vi "RecordAV_CB.vi"(4 "ErrorIn":errorcluster, 5 "DataFolder":string="00000000-000000", 6 "Source":enum16{"AI0", "SoundCard"}(ring), 7 "Mode":T2(ring)=enum."Close") -> (0 "ErrorOut":errorcluster={"status"=FALSE, "code"=209801, "source"="Send2Grapevine32.vi"})   [LabVIEW 2013]
doc: "The Low-Level Grab VI configures the number of buffers to use for the acquisition and configures an event callback to handle every other acquired image. A grab is appropriate for high-speed applications in which you need to process only one image at a time."
uses:
  <vilib>/vision/Image Controls.llb/IMAQ Image.ctl
  <vilib>/userdefined/High Color/IMAQdx.ctl
  <vilib>/vision/Avi.llb/IMAQ AVI2 Refnum.ctl
  <vilib>/sound2/lvsound2.llb/Sound File Refnum.ctl
  <vilib>/sound2/lvsound2.llb/Sound Input Task ID.ctl
  <vilib>/vision/driver/IMAQdx.llb/IMAQdx Acquisition Mode.ctl
  <vilib>/sound2/lvsound2.llb/Sound Data Format.ctl
  <vilib>/sound2/lvsound2.llb/Sampling Mode.ctl
  <vilib>/vision/driver/IMAQdx.llb/IMAQdx Buffer Number Mode.ctl
  <vilib>/DAQmx/read.llb/DAQmx Read (Analog 2D DBL NChan NSamp).vi
  <vilib>/sound2/lvsound2.llb/Sound File Write Open.vi
  <vilib>/sound2/lvsound2.llb/Sound File Write (DBL Single).vi
  Globals.vi
  <vilib>/DAQmx/miscellaneous.llb/DAQmx Fill In Error Info.vi
  <vilib>/sound2/lvsound2.llb/Sound Input Read (SGL).vi
  <vilib>/vision/driver/NI_Vision_Acquisition_Software.lvlib
  <resource>/objmgr/imaqdx.rc
panel:
  out "iSource":enum16{"AI0", "SoundCard"}(ring)=enum."SoundCard"
  out "AudID":T1=1 format="%.0x"
  out "VidTask":T3="cam1"
  out "AudTask":refnum<k21>
  out "WAVRef":T4
  out "AVIRef":T5
  out "FrmEvnt":refnum<event-registration>
  out "BufferImg":T6
  out "StopAud":bool
  out "StopVid":bool
  out "StitchResult":string="ffmpeg version N-51683-g9dc88ac Copyright (c) 2000-2013 the FFmpeg developers\r\n  built on Apr  8 2013 21:24:37 with gcc 4.8.0 (GCC)\r\n  configuration: --enable-gpl --enable-version3 --disable-w32threads --enable-avisynth --enable-bzlib --enable-fontconfig --enable-frei0r --enable-gnutls --enable-iconv --enable-libass --enable-libbluray --enable-libcaca --enable-libfreetype --enable-libgsm --enable-libilbc --enable-libmp3lame --enable-libopencore-amrnb --enable-libopencore-amrwb --enable-libopenjpeg --enable-libopus --enable-librtmp --enable-libschroedinger --enable-libsoxr --enable-libspeex --enable-libtheora --enable-libtwolame --enable-libvo-aacenc --enable-libvo-amrwbenc --enable-libvorbis --enable-libvpx --enable-libx264 --enable-libxavs --enable-libxvid --enable-zlib\r\n  libavutil      52. 25.100 / 52. 25.100\r\n  libavcodec     55.  2.100 / 55.  2.100\r\n  libavformat    55.  1.100 / 55.  1.100\r\n  libavdevice    55.  0.100 / 55.  0.100\r\n  libavfilter     3. 49.101 /  3. 49.101\r\n  libswscale      2.  2.100 /  2.  2.100\r\n  libswresample   0. 17.102 /  0. 17.102\r\n  libpostproc    52.  2.100 / 52.  2.100\r\nInput #0, avi, from 'D:\\20140505-075330\\20140505-075330.avi':\r\n  Duration: 00:00:50.56, start: 0.000000, bitrate: 1016 kb/s\r\n    Stream #0:0: Video: mpeg4 (Simple Profile) (XVID / 0x44495658), yuv420p, 1280x720 [SAR 1:1 DAR 16:9], 25 tbr, 25 tbn, 25 tbc\r\n[wav @ 0000000003b3a5a0] max_analyze_duration 5000000 reached at 5015510 microseconds\r\nGuessed Channel Layout for  Input Stream #1.0 : mono\r\nInput #1, wav, from 'D:\\20140505-075330\\20140505-075330.wav':\r\n  Duration: 00:00:50.00, bitrate: 705 kb/s\r\n    Stream #1:0: Audio: pcm_s16le ([1][0][0][0] / 0x0001), 44100 Hz, mono, s16, 705 kb/s\r\nOutput #0, avi, to 'D:\\20140505-075330\\20140505-075330_Mixed.avi':\r\n  Metadata:\r\n    ISFT            : Lavf55.1.100\r\n    Stream #0:0: Video: mpeg4 (XVID / 0x44495658), yuv420p, 1280x720 [SAR 1:1 DAR 16:9], q=2-31, 25 tbn, 25 tbc\r\n    Stream #0:1: Audio: mp3 (U[0][0][0] / 0x0055), 44100 Hz, mono, s16p\r\nStream mapping:\r\n  Stream #0:0 -> #0:0 (copy)\r\n  Stream #1:0 -> #0:1 (pcm_s16le -> libmp3lame)\r\nPress [q] to stop, [?] for help\r\nframe=  184 fps=0.0 q=-1.0 size=     434kB time=00:00:07.36 bitrate= 482.9kbits/s    \rframe=  738 fps=726 q=-1.0 size=    4068kB time=00:00:29.52 bitrate=1129.0kbits/s    \rframe= 1264 fps=1015 q=-1.0 Lsize=    6718kB time=00:00:50.56 bitrate=1088.5kbits/s    \r\r\nvideo:6241kB audio:391kB subtitle:0 global headers:0kB muxing overhead 1.308708%\r\n"
  out "WAVName":path=path "D:/20140505-075330/20140505-075330.wav"
  out "AVIName":path=path "D:/20140505-075330/20140505-075330.avi"
  out "FrameRate":dbl=25.0
  out "WAVChart":dbl[](graph)=[0.01885986328125, 0.02471923828125, 0.026458740234375, 0.019622802734375, 0.015625, 0.016571044921875, 0.017852783203125, 0.016937255859375, 0.02349853515625, 0.0262451171875, 0.021697998046875, 0.01995849609375, 0.013427734375, 0.008819580078125, 0.013916015625, 0.016693115234375, 0.0172119140625, 0.023468017578125, 0.0235595703125, 0.018890380859375, 0.022369384765625, 0.022003173828125, 0.019378662109375, 0.017578125, 0.0115966796875, 0.011688232421875, 0.011016845703125, 0.007659912109375, 0.012359619140625, 0.015167236328125, 0.010162353515625, 0.00787353515625, 0.010009765625, 0.01434326171875, 0.018524169921875, 0.019012451171875, 0.019317626953125, 0.019500732421875, 0.021514892578125, 0.021514892578125, 0.0233154296875, 0.02276611328125, 0.0174560546875, 0.018585205078125, 0.019439697265625, 0.01959228515625, 0.0185546875, 0.015594482421875, 0.01593017578125, 0.0162353515625, 0.013427734375, 0.01519775390625, 0.005340576171875, 0.008026123046875, 0.00811767578125, 0.004669189453125, 0.008148193359375, 0.00384521484375, 0.007598876953125, 0.007354736328125, 0.009735107421875, 0.01580810546875, 0.01385498046875, 0.014923095703125, 0.00830078125, 0.005096435546875, 0.008941650390625, 0.01416015625, 0.01220703125, 0.0140380859375, 0.01275634765625, 0.006439208984375, 0.007049560546875, 0.006134033203125, -0.000457763671875, 0.003326416015625, 0.0081787109375, 0.009124755859375, 0.013458251953125, 0.014007568359375, 0.014312744140625, 0.006011962890625, 0.00238037109375, 0.010284423828125, 0.011962890625, 0.009857177734375, 0.00909423828125, 0.016448974609375, 0.01885986328125, 0.01190185546875, 0.010955810546875, 0.01019287109375, 0.00152587890625, 0.00762939453125, 0.008270263671875, 0.00604248046875, 0.010589599609375, 0.0037841796875, 0.0050048828125, 0.007080078125, 0.004669189453125, 0.0064697265625, 0.01068115234375, 0.009521484375, 0.002532958984375, -0.000518798828125, 0.005035400390625, 0.0042724609375, 0.00164794921875, 0.0001220703125, -0.002716064453125, -0.00164794921875, -0.007232666015625, -0.01153564453125, -0.005889892578125, -0.00341796875, -0.008514404296875, -0.007415771484375, -0.00726318359375, -0.007781982421875, -0.009918212890625, -0.010772705078125, -0.00628662109375, -0.001373291015625, -0.0008544921875, -0.003997802734375, 0.003021240234375, 0.003082275390625, 0.000640869140625, 0.00250244140625, 0.002960205078125, 0.00115966796875, 0.000579833984375, -0.002166748046875, -0.00115966796875, -0.006591796875, -0.0128173828125, -0.013275146484375, -0.0157470703125, -0.016204833984375, -0.013885498046875, -0.01531982421875, -0.00897216796875, -0.00762939453125, -0.00738525390625, -0.00311279296875, -0.002166748046875, 0.000244140625, -0.003509521484375, -0.003662109375, 0.001220703125, 0.001251220703125, 0.0001220703125, -0.003692626953125, -0.003997802734375, -0.004364013671875, -9.1552734375e-05, 0.00341796875, 0.000457763671875, -0.000274658203125, -0.0006103515625, 0.00543212890625, 0.001312255859375, 0.003662109375, 0.009765625, 0.004852294921875, 0.003997802734375, 0.00189208984375, -0.000213623046875, -0.006500244140625, -0.006744384765625, -0.0120849609375, -0.012359619140625, -0.003631591796875, -0.005645751953125, -0.0028076171875, 0.00286865234375, -0.00311279296875, -0.005279541015625, 0.001922607421875, -0.003753662109375, -0.000335693359375, -0.00299072265625, 0.001556396484375, 0.00299072265625, 0.006317138671875, 0.006622314453125, -0.003692626953125, -0.007110595703125, 0.001190185546875, -0.002288818359375, 0.00030517578125, 0.007720947265625, 0.003692626953125, 0.006011962890625, 0.007904052734375, 0.0115966796875, 0.01513671875, 0.00421142578125, 0.00299072265625, 0.002532958984375, 0.0009765625, 0.0018310546875, 0.001556396484375, 0.00640869140625, 0.008148193359375, 0.011962890625, 0.01416015625, 0.01055908203125, 0.0126953125, 0.006500244140625, 0.00958251953125, 0.009613037109375, 0.00921630859375, 0.007049560546875, 0.00927734375, 0.011871337890625, 0.015655517578125, 0.0146484375, 0.011627197265625, 0.0162353515625, 0.007965087890625, 0.00146484375, 0.004425048828125, 0.007415771484375, 0.007598876953125, 0.011810302734375, 0.01324462890625, 0.016357421875, 0.0126953125, 0.012451171875, 0.01763916015625, 0.0196533203125, 0.019775390625, 0.021453857421875, 0.025848388671875, 0.023468017578125, 0.01934814453125, 0.019073486328125, 0.020355224609375, 0.021270751953125, 0.024139404296875, 0.02545166015625, 0.0255126953125, 0.027862548828125, 0.027435302734375, 0.030487060546875, 0.029052734375, 0.032196044921875, 0.030120849609375, 0.035552978515625, 0.026611328125, 0.025787353515625, 0.030303955078125, 0.021270751953125, 0.027099609375, 0.032379150390625, 0.03143310546875, 0.02508544921875, 0.03118896484375, 0.029510498046875, 0.0311279296875, 0.03460693359375, 0.0340576171875, 0.027435302734375, 0.03076171875, 0.031707763671875, 0.029815673828125, 0.0341796875, 0.039337158203125, 0.0396728515625, 0.039459228515625, 0.031463623046875, 0.025482177734375, 0.03057861328125, 0.031707763671875, 0.03253173828125, 0.035308837890625, 0.0355224609375, 0.035369873046875, 0.02996826171875, 0.0267333984375, 0.025665283203125, 0.024688720703125, 0.029754638671875, 0.023681640625, 0.02490234375, 0.026458740234375, 0.025726318359375, 0.03436279296875, 0.028411865234375, 0.0225830078125, 0.02349853515625, 0.021270751953125, 0.02691650390625, 0.02520751953125, 0.023101806640625, 0.020782470703125, 0.0198974609375, 0.024200439453125, 0.021148681640625, 0.023406982421875, 0.028289794921875, 0.02862548828125, 0.03240966796875, 0.025634765625, 0.030120849609375, 0.029998779296875, 0.02752685546875, 0.033660888671875, 0.028167724609375, 0.032073974609375, 0.033233642578125, 0.02862548828125, 0.029876708984375, 0.02667236328125, 0.02392578125, 0.02764892578125, 0.026275634765625, 0.023468017578125, 0.031158447265625, 0.0306396484375, 0.022125244140625, 0.022430419921875, 0.025054931640625, 0.02337646484375, 0.025299072265625, 0.02777099609375, 0.03326416015625, 0.02777099609375, 0.025390625, 0.028778076171875, 0.02239990234375, 0.01837158203125, 0.021148681640625, 0.021514892578125, 0.018218994140625, 0.01593017578125, 0.017547607421875, 0.018524169921875, 0.01739501953125, 0.01922607421875, 0.016632080078125, 0.010772705078125, 0.013519287109375, 0.011383056640625, 0.013671875, 0.017242431640625, 0.021636962890625, 0.01922607421875, 0.01593017578125, 0.016571044921875, 0.015777587890625, 0.016693115234375, 0.011260986328125, 0.005828857421875, 0.0068359375, 0.001739501953125, 0.00518798828125, 0.006591796875, 0.00286865234375, 0.015289306640625, 0.011383056640625, 0.01031494140625, 0.00927734375, 0.009307861328125, 0.011199951171875, 0.010894775390625, 0.006927490234375, 0.0115966796875, 0.004638671875, 0.004425048828125, 0.003631591796875, 0.007659912109375, 0.0086669921875, 0.00616455078125, 0.003509521484375, -0.000518798828125, 0.0001220703125, -0.001708984375, -0.0015869140625, 0.002349853515625, 0.0089111328125, 0.007171630859375, 0.0072021484375, 0.004791259765625, 0.00341796875, 0.001068115234375, 0.00341796875, 0.00445556640625, 0.008056640625, 0.009246826171875, 0.011077880859375, 0.006195068359375, 0.005340576171875, 0.00244140625, 0.006561279296875, 0.016021728515625, 0.011322021484375, 0.0079345703125, 0.006622314453125, 0.01080322265625, 0.009796142578125, 0.0028076171875, 0.00439453125, 0.00048828125, 0.0052490234375, 0.0025634765625, 0.00396728515625, 0.0057373046875, 0.00860595703125, 0.00701904296875, 0.0020751953125, -0.00189208984375, -0.001861572265625, 0.00091552734375, -0.00762939453125, -0.0074462890625, -0.0054931640625, 0.0010986328125, 0.00421142578125, 0.001800537109375, 0.007232666015625, -0.001190185546875, 9.1552734375e-05, -0.0078125, -0.010833740234375, -0.0068359375, -0.0054931640625, -0.004791259765625, -0.011016845703125, -0.009765625, -0.007720947265625, -0.00384521484375, -0.011260986328125, -0.00848388671875, -0.000152587890625, -0.00030517578125, -0.00177001953125, -0.0052490234375, -0.00994873046875, -0.001617431640625, -0.00567626953125, -0.008209228515625, -0.004638671875, -0.0057373046875, -0.0067138671875, -0.01080322265625, -0.008544921875, -0.0120849609375, -0.009857177734375, -0.01409912109375, -0.0184326171875, -0.022003173828125, -0.023101806640625, -0.02197265625, -0.021942138671875, -0.018035888671875, -0.016632080078125, -0.025726318359375, -0.032623291015625, -0.02557373046875, -0.03179931640625, -0.020660400390625, -0.017578125, -0.01641845703125, -0.017852783203125, -0.02423095703125, -0.030609130859375, -0.03009033203125, -0.027862548828125, -0.031646728515625, -0.03076171875, -0.0225830078125, -0.015472412109375, -0.018341064453125, -0.02520751953125, -0.032958984375, -0.034759521484375, -0.034637451171875, -0.033233642578125, -0.031768798828125, -0.025238037109375, -0.02752685546875, -0.03057861328125, -0.0286865234375, -0.03204345703125, -0.02850341796875, -0.020965576171875, -0.022735595703125, -0.02435302734375, -0.024383544921875, -0.02496337890625, -0.01910400390625, -0.0230712890625, -0.0225830078125, -0.02435302734375, -0.027984619140625, -0.027740478515625, -0.026153564453125, -0.03021240234375, -0.030792236328125, -0.0277099609375, -0.0250244140625, -0.02239990234375, -0.025146484375, -0.029571533203125, -0.022491455078125, -0.02587890625, -0.02081298828125, -0.024688720703125, -0.026885986328125, -0.026214599609375, -0.025482177734375, -0.027374267578125, -0.03387451171875, -0.03570556640625, -0.0379638671875, -0.03662109375, -0.034637451171875, -0.03826904296875, -0.0408935546875, -0.037384033203125, -0.038177490234375, -0.039337158203125, -0.03564453125, -0.02972412109375, -0.02410888671875, -0.01873779296875, -0.02288818359375, -0.02679443359375, -0.03839111328125, -0.0316162109375, -0.029449462890625, -0.02972412109375, -0.03564453125, -0.034332275390625, -0.038665771484375, -0.044525146484375, -0.040374755859375, -0.039031982421875, -0.03741455078125, -0.039703369140625, -0.0386962890625, -0.036834716796875, -0.03521728515625, -0.033905029296875, -0.02984619140625, -0.035430908203125, -0.032440185546875, -0.029022216796875, -0.024688720703125, -0.024139404296875, -0.027099609375, -0.027313232421875, -0.02496337890625, -0.02203369140625, -0.0244140625, -0.021240234375, -0.02392578125, -0.020782470703125, -0.01873779296875, -0.0208740234375, -0.0208740234375, -0.022491455078125, -0.01806640625, -0.0216064453125, -0.017181396484375, -0.01397705078125, -0.01556396484375, -0.009979248046875, -0.016693115234375, -0.01068115234375, -0.016754150390625, -0.01959228515625, -0.016143798828125, -0.02447509765625, -0.029266357421875, -0.026947021484375, -0.02496337890625, -0.0345458984375, -0.027618408203125, -0.0318603515625, -0.028656005859375, -0.02685546875, -0.025634765625, -0.02392578125, -0.026031494140625, -0.014617919921875, -0.018585205078125, -0.021697998046875, -0.019317626953125, -0.02044677734375, -0.0184326171875, -0.018951416015625, -0.022125244140625, -0.019073486328125, -0.02203369140625, -0.0224609375, -0.02166748046875, -0.019073486328125, -0.015411376953125, -0.016448974609375, -0.023834228515625, -0.021728515625, -0.016387939453125, -0.009490966796875, -0.012542724609375, -0.0169677734375, -0.017822265625, -0.02105712890625, -0.017913818359375, -0.016815185546875, -0.01983642578125, -0.0179443359375, -0.0123291015625, -0.01129150390625, -0.01324462890625, -0.015869140625, -0.01385498046875, -0.016387939453125, -0.015655517578125, -0.0181884765625, -0.017578125, -0.013092041015625, -0.008331298828125, -0.007781982421875, -0.00439453125, -0.007080078125, -0.010223388671875, -0.01239013671875, -0.014923095703125, -0.01080322265625, -0.001983642578125, -0.0074462890625, -0.017791748046875, -0.023040771484375, -0.02978515625, -0.0267333984375, -0.0224609375, -0.017120361328125, -0.024871826171875, -0.01788330078125, -0.012298583984375, -0.011566162109375, -0.00726318359375, -0.00457763671875, -0.00299072265625, 0.00146484375, -0.0037841796875, -0.008819580078125, -0.0076904296875, -0.006256103515625, 0.001373291015625, -0.001708984375, -0.00335693359375, 0.001953125, 0.005859375, 0.00396728515625, 0.007110595703125, 0.011993408203125, 0.005828857421875, 0.00677490234375, 0.000244140625, 0.008575439453125, 0.0098876953125, 0.003875732421875, 0.0067138671875, 0.000946044921875, 0.00274658203125, 0.001800537109375, 0.00506591796875, 0.006072998046875, -0.006103515625, -0.00909423828125, -0.003936767578125, -0.001861572265625, -0.002777099609375, 0.001495361328125, 0.0006103515625, -0.003265380859375, -0.0003662109375, 0.00128173828125, 0.0010986328125, 0.002655029296875, -0.005615234375, -0.01275634765625, -0.00775146484375, -0.004913330078125, -0.004119873046875, -0.00506591796875, -9.1552734375e-05, 0.003204345703125, -0.002410888671875, -0.001800537109375, 0.001312255859375, 0.003173828125, -0.002899169921875, -0.004608154296875, 0.002593994140625, -0.002685546875, -0.00762939453125, -0.0028076171875, -0.006805419921875, -0.0146484375, -0.009979248046875, -0.00177001953125, 0.00286865234375, -0.0091552734375, -0.01495361328125, -0.01080322265625, -0.009368896484375, 0.0023193359375, -0.0010986328125, -0.001678466796875, -0.00177001953125, -0.006134033203125, -0.004730224609375, -0.00921630859375, -0.00909423828125, -0.0108642578125, -0.017181396484375, -0.015289306640625, -0.01458740234375, -0.013336181640625, -0.0057373046875, -0.004852294921875, -0.005645751953125, -0.0050048828125, -0.006500244140625, -0.00927734375, -0.012908935546875, -0.014404296875, -0.0155029296875, -0.0115966796875, -0.009796142578125, -0.01202392578125, -0.018157958984375, -0.021240234375, -0.015533447265625, -0.01629638671875, -0.01318359375, -0.015594482421875, -0.020721435546875, -0.017974853515625, -0.02056884765625, -0.02264404296875, -0.01654052734375, -0.01702880859375, -0.0146484375, -0.013275146484375, -0.023040771484375, -0.015960693359375, -0.013092041015625, -0.011077880859375, -0.009063720703125, -0.01727294921875, -0.018035888671875, -0.01580810546875, -0.011932373046875, -0.01287841796875, -0.003692626953125, -0.015167236328125, -0.014068603515625, -0.01666259765625, -0.0211181640625, -0.01812744140625, -0.013336181640625, -0.01519775390625, -0.0093994140625, -0.012847900390625, -0.0208740234375, -0.01300048828125, -0.006988525390625, -0.006072998046875, -0.011199951171875, -0.01263427734375, -0.01263427734375, -0.015625, -0.01055908203125, -0.00372314453125, -0.001312255859375, 0.001861572265625, -6.103515625e-05, -0.00311279296875, -0.001251220703125, -0.006500244140625, -0.00665283203125, 0.000823974609375, 0.001190185546875, 0.004486083984375, -0.004638671875, -0.00250244140625, -0.000518798828125, 0.001739501953125, 0.010955810546875, 0.00384521484375, -0.002349853515625, -0.00128173828125, -0.002227783203125, -0.005157470703125, -0.003204345703125, -0.00482177734375, -0.006072998046875, -0.001312255859375, -0.00018310546875, 0.0001220703125, -0.000274658203125, 0.003753662109375, 0.0103759765625, 0.009063720703125, 0.01324462890625, 0.019989013671875, 0.01324462890625, 0.015350341796875, 0.017791748046875, 0.019744873046875, 0.0157470703125, 0.007049560546875, 0.01263427734375, 0.0111083984375, 0.009002685546875, 0.01141357421875, 0.016632080078125, 0.012847900390625, 0.007568359375, 0.0042724609375, -0.00372314453125, -0.011383056640625, 0.00128173828125, 0.014312744140625, 0.016082763671875, 0.021697998046875, 0.020172119140625, 0.021575927734375, 0.02032470703125, 0.02215576171875, 0.02471923828125, 0.0302734375, 0.02752685546875, 0.02667236328125, 0.026580810546875, 0.0250244140625, 0.027557373046875, 0.020172119140625, 0.0247802734375, 0.02978515625, 0.030120849609375, 0.03131103515625, 0.031524658203125, 0.032257080078125, 0.0286865234375, 0.03033447265625, 0.0279541015625, 0.03582763671875, 0.036285400390625, 0.03515625, 0.028656005859375, 0.0311279296875, 0.033599853515625, 0.03582763671875, 0.028839111328125, 0.02947998046875, 0.0306396484375, 0.025146484375, 0.020843505859375, 0.027679443359375, 0.028045654296875, 0.02532958984375, 0.024017333984375, 0.02410888671875, 0.032073974609375, 0.018951416015625, 0.02801513671875, 0.0318603515625, 0.02587890625, 0.02825927734375, 0.025421142578125, 0.033203125, 0.03515625, 0.0362548828125, 0.030975341796875, 0.034332275390625, 0.02392578125, 0.027191162109375, 0.03472900390625, 0.03515625, 0.02813720703125, 0.0291748046875, 0.028717041015625, 0.027099609375, 0.02874755859375, 0.02203369140625, 0.019805908203125, 0.0179443359375, 0.0289306640625, 0.023773193359375, 0.017059326171875, 0.020904541015625, 0.0262451171875, 0.022979736328125, 0.021453857421875, 0.024017333984375, 0.02056884765625, 0.022430419921875, 0.02081298828125, 0.021759033203125, 0.026611328125, 0.033660888671875, 0.027374267578125, 0.02435302734375, 0.0185546875, 0.018096923828125, 0.023223876953125, 0.01654052734375, 0.015899658203125, 0.009490966796875, 0.00897216796875, 0.00933837890625, 0.013763427734375, 0.01470947265625, 0.021392822265625, 0.0238037109375, 0.022979736328125, 0.025665283203125, 0.0169677734375, 0.0174560546875, 0.015472412109375, 0.012786865234375, 0.011688232421875, 0.0103759765625, 0.00640869140625, 0.0113525390625, 0.0142822265625, 0.012603759765625, 0.0142822265625, 0.016815185546875, 0.020782470703125, 0.012237548828125, 0.008392333984375, 0.017578125, 0.019775390625, 0.026336669921875, 0.02557373046875, 0.019317626953125, 0.015380859375, 0.0196533203125, 0.01812744140625, 0.020050048828125, 0.015045166015625, 0.01416015625, 0.01129150390625, 0.00885009765625, 0.00799560546875, 0.01055908203125, 0.0107421875, 0.0164794921875, 0.0133056640625, 0.0064697265625, 0.0089111328125, 0.0069580078125, 0.0064697265625, 0.001220703125, -0.003082275390625, -0.0028076171875, -9.1552734375e-05, 0.00201416015625, -0.000946044921875, -0.001495361328125, 0.000579833984375, 0.003265380859375, 0.00390625, 0.005889892578125, 0.002685546875, -0.000732421875, 0.004058837890625, 0.0023193359375, 0.008544921875, 0.00250244140625, -0.000885009765625, -0.00244140625, -0.004608154296875, -0.002288818359375, -0.0050048828125, -0.000885009765625, -0.0013427734375, 0.001800537109375, 0.001678466796875, -0.005279541015625, 0.00506591796875, 0.002899169921875, 0.003662109375, 0.0087890625, 0.011474609375, 0.01422119140625, 0.01055908203125, 0.011444091796875, 0.012359619140625, 0.001190185546875, 0.0054931640625, 0.007598876953125, 0.01025390625, 0.01300048828125, 0.008575439453125, 0.007659912109375, 0.00897216796875, 0.014892578125, 0.01226806640625, 0.014434814453125, 0.022003173828125, 0.02056884765625, 0.022705078125, 0.02532958984375, 0.02154541015625, 0.02130126953125, 0.01788330078125, 0.016845703125, 0.018524169921875, 0.015167236328125, 0.01947021484375, 0.017578125, 0.01470947265625, 0.015533447265625, 0.015594482421875, 0.00836181640625, 0.0164794921875, 0.017608642578125, 0.012481689453125, 0.01287841796875, 0.01123046875, 0.010986328125, 0.01324462890625, 0.015655517578125, 0.01287841796875, 0.0107421875, 0.012908935546875, 0.00885009765625, 0.00201416015625, 0.008026123046875, 0.00994873046875, 0.011444091796875, 0.010894775390625, 0.01385498046875, 0.0174560546875, 0.014495849609375, 0.009246826171875, 0.00982666015625, 0.010406494140625, 0.015411376953125, 0.01507568359375, 0.0067138671875, 0.009521484375, 0.011322021484375, 0.00811767578125, -0.002410888671875, 0.00299072265625, -0.004852294921875, 0.0032958984375, 0.0032958984375, 6.103515625e-05, 0.00152587890625, 0.003082275390625, 0.011627197265625, 0.013458251953125, 0.01239013671875, 0.015777587890625, 0.023406982421875, 0.027923583984375, 0.024139404296875, 0.020721435546875, 0.022308349609375, 0.026519775390625, 0.019256591796875, 0.013214111328125, 0.0146484375, 0.015777587890625, 0.02001953125, 0.0150146484375, 0.01055908203125, 0.00897216796875, 0.00823974609375, 0.0013427734375, 0.005615234375, -0.00225830078125, -0.008087158203125, 0.005950927734375, 0.00762939453125, 0.003326416015625, 0.009002685546875, 0.006744384765625, 0.0101318359375, 0.00732421875, 0.004425048828125, 0.01068115234375, 0.001251220703125, 0.008758544921875, 0.018218994140625, 0.013885498046875, 0.014617919921875, 0.011383056640625, 0.01373291015625, 0.0115966796875, 0.00567626953125, 0.002716064453125, -0.000823974609375, 0.0025634765625, 0.0028076171875, 0.002044677734375, -0.000335693359375, 0.0029296875, 0.002655029296875, 0.002349853515625, 0.001678466796875, 0.00433349609375, 0.011871337890625, 0.006744384765625, 0.001129150390625, 0.000640869140625, -0.00042724609375, -0.007781982421875, -0.00433349609375, -0.002166748046875, 0.00189208984375, 0.000823974609375, -0.001922607421875, -0.000152587890625, -0.001007080078125, -0.005035400390625, -0.006439208984375, -0.00799560546875, -0.0150146484375, -0.017822265625, -0.02020263671875, -0.012542724609375, -0.01116943359375, -0.012298583984375, -0.017974853515625, -0.011810302734375, -0.009674072265625, -0.01446533203125, -0.0096435546875, -0.017852783203125, -0.0228271484375, -0.024505615234375, -0.022064208984375, -0.01568603515625, -0.01495361328125, -0.017242431640625, -0.014862060546875, -0.011871337890625, -0.009979248046875, -0.007965087890625, -0.007598876953125, -0.00628662109375, -0.009613037109375, -0.00982666015625, -0.0140380859375, -0.013275146484375, -0.016510009765625, -0.02313232421875, -0.019744873046875, -0.02117919921875, -0.024261474609375, -0.023406982421875, -0.025634765625, -0.026123046875, -0.029937744140625, -0.0272216796875, -0.025054931640625, -0.0198974609375, -0.020263671875, -0.022705078125, -0.0177001953125, -0.018585205078125, -0.020751953125, -0.01678466796875, -0.017181396484375, -0.016937255859375, -0.01995849609375, -0.014312744140625, -0.015350341796875, -0.016815185546875, -0.014129638671875, -0.02496337890625, -0.019317626953125, -0.023193359375, -0.017059326171875, -0.015533447265625, -0.020843505859375, -0.01788330078125, -0.021575927734375, -0.016876220703125, -0.0162353515625, -0.01556396484375, -0.02313232421875, -0.017822265625, -0.011871337890625, -0.0125732421875, -0.01348876953125, -0.014312744140625, -0.00909423828125, -0.009063720703125, -0.010345458984375, -0.00726318359375, -0.01397705078125, -0.009490966796875, -0.00982666015625, -0.007598876953125, -0.00421142578125, -0.00067138671875, 0.001953125, 0.001556396484375, 0.001220703125, -0.009185791015625, -0.013336181640625, -0.01556396484375, -0.01116943359375, -0.0096435546875, -0.010162353515625, -0.011749267578125, -0.012359619140625, -0.009124755859375, -0.009857177734375, -0.011474609375, -0.007568359375, -0.0068359375, -0.0062255859375, -0.00482177734375, -0.010467529296875, -0.0078125, -0.00750732421875, -0.01434326171875, -0.01361083984375, -0.0181884765625, -0.020782470703125, -0.007568359375, -0.006988525390625, -0.006622314453125, -0.001861572265625, -0.00128173828125, -0.0115966796875, -0.005401611328125, -0.004974365234375, -0.0084228515625, -0.011383056640625, -0.0118408203125, -0.008148193359375, -0.006256103515625, -0.001861572265625, 0.004302978515625, 0.004913330078125, 0.006195068359375, 0.00897216796875, 0.003753662109375, 0.00360107421875, -0.00201416015625, -0.001190185546875, -0.0030517578125, -0.0067138671875, -0.00469970703125, -0.005828857421875, -0.005645751953125, 0.001708984375, 0.002960205078125, 0.005767822265625, 0.001983642578125, 0.00048828125, -0.00103759765625, -0.001556396484375, 0.0, 0.007659912109375, 0.01202392578125, 0.010986328125, 0.0059814453125, 0.007354736328125, 0.01275634765625, 0.010009765625, 0.008880615234375, 0.008544921875, 0.007354736328125, 0.001800537109375, 0.00115966796875, -0.002410888671875, 0.009063720703125, 0.01190185546875, 0.012908935546875, 0.010650634765625, 0.004974365234375, 0.01251220703125, 0.012603759765625, 0.007110595703125, 0.00860595703125, 0.017303466796875, 0.01348876953125, 0.01556396484375, 0.0159912109375, 0.0147705078125, 0.01861572265625, 0.014068603515625, 0.0167236328125, 0.015533447265625, 0.0198974609375, 0.019866943359375, 0.015350341796875, 0.0079345703125, 0.0091552734375, 0.00921630859375, 0.011077880859375, 0.00738525390625, 0.008544921875, 0.01690673828125, 0.01513671875, 0.010009765625, 0.0107421875, 0.009674072265625, 0.0142822265625, 0.015899658203125, 0.012359619140625, 0.0203857421875, 0.02166748046875, 0.02032470703125, 0.02069091796875, 0.018280029296875, 0.010772705078125, 0.0057373046875, 0.013519287109375, 0.017242431640625, 0.011383056640625, 0.0142822265625, 0.013824462890625, 0.011962890625, 0.010284423828125, 0.0089111328125, 0.011993408203125, 0.0103759765625, -3.0517578125e-05, -0.00640869140625, -0.00506591796875, -0.00701904296875, -0.003143310546875, 0.0037841796875, 0.008209228515625, 0.00518798828125, 0.00506591796875, 0.006591796875, 0.00701904296875, 0.00567626953125, 0.011383056640625, 0.00543212890625, 0.001556396484375, 0.009185791015625, 0.00628662109375, 0.009521484375, 0.01324462890625, 0.0198974609375, 0.01837158203125, 0.017669677734375, 0.0103759765625, 0.013214111328125, 0.015594482421875, 0.014495849609375, 0.013092041015625, 0.010711669921875, 0.006195068359375, 0.0054931640625, 0.012969970703125, 0.01123046875, 0.017974853515625, 0.015106201171875, 0.011505126953125, 0.009307861328125, 0.024322509765625, 0.023284912109375, 0.01983642578125, 0.025726318359375, 0.030059814453125, 0.0242919921875, 0.02655029296875, 0.03326416015625, 0.023712158203125, 0.02374267578125, 0.022552490234375, 0.0157470703125, 0.020782470703125, 0.022064208984375, 0.022430419921875, 0.0272216796875, 0.02301025390625, 0.019744873046875, 0.018768310546875, 0.0240478515625, 0.029876708984375, 0.032196044921875, 0.030975341796875, 0.026458740234375, 0.025421142578125, 0.023529052734375, 0.024505615234375, 0.021697998046875, 0.018768310546875, 0.0145263671875, 0.01544189453125, 0.0244140625, 0.0198974609375, 0.017578125, 0.021148681640625, 0.01885986328125, 0.0191650390625, 0.018890380859375, 0.02740478515625, 0.018646240234375, 0.02069091796875, 0.025787353515625, 0.02423095703125, 0.0245361328125, 0.022796630859375, 0.01898193359375, 0.01727294921875, 0.021514892578125, 0.014739990234375, 0.01812744140625, 0.023651123046875, 0.020263671875, 0.01995849609375, 0.01971435546875, 0.021331787109375, 0.013336181640625, 0.01605224609375, 0.020111083984375, 0.0228271484375, 0.01959228515625, 0.0181884765625, 0.02130126953125, 0.00885009765625, 0.0120849609375, 0.012786865234375, 0.01593017578125, 0.021728515625, 0.021636962890625, 0.02227783203125, 0.017791748046875, 0.01885986328125, 0.025177001953125, 0.027557373046875, 0.019287109375, 0.01025390625, 0.01348876953125, 0.014129638671875, 0.02435302734375, 0.026336669921875, 0.02685546875, 0.0263671875, 0.029052734375, 0.03204345703125, 0.026580810546875, 0.033050537109375, 0.03021240234375, 0.02557373046875, 0.02392578125, 0.027801513671875, 0.0362548828125, 0.036041259765625, 0.03271484375, 0.03167724609375, 0.0325927734375, 0.038818359375, 0.036163330078125, 0.037017822265625, 0.030364990234375, 0.02996826171875, 0.029754638671875, 0.02813720703125, 0.021087646484375, 0.02264404296875, 0.020782470703125, 0.02197265625, 0.026580810546875, 0.020111083984375, 0.023834228515625, 0.02264404296875, 0.018157958984375, 0.026123046875, 0.027130126953125, 0.027618408203125, 0.031829833984375, 0.030487060546875, 0.027587890625, 0.025115966796875, 0.02667236328125, 0.0299072265625, 0.030426025390625, 0.0299072265625, 0.033599853515625, 0.035491943359375, 0.0390625, 0.035369873046875, 0.029266357421875, 0.022247314453125, 0.029083251953125, 0.022186279296875, 0.017181396484375, 0.02008056640625, 0.02447509765625, 0.027984619140625, 0.020782470703125, 0.0203857421875, 0.02197265625, 0.02520751953125, 0.018524169921875, 0.01922607421875, 0.02557373046875, 0.020599365234375, 0.025421142578125, 0.02606201171875, 0.026885986328125, 0.025970458984375, 0.0262451171875, 0.024200439453125, 0.0257568359375, 0.024078369140625, 0.02227783203125, 0.027923583984375, 0.0250244140625, 0.01995849609375, 0.022369384765625, 0.020538330078125, 0.021026611328125, 0.02734375, 0.0316162109375, 0.0347900390625, 0.0272216796875, 0.03057861328125, 0.034454345703125, 0.0289306640625, 0.035491943359375, 0.033538818359375, 0.023651123046875, 0.025848388671875, 0.0223388671875, 0.018646240234375, 0.01934814453125, 0.02130126953125, 0.01800537109375, 0.01824951171875, 0.01837158203125, 0.017242431640625, 0.021148681640625, 0.02520751953125, 0.02197265625, 0.021270751953125, 0.01971435546875, 0.0244140625, 0.02313232421875, 0.0244140625, 0.0272216796875, 0.0302734375, 0.023895263671875, 0.027374267578125, 0.031097412109375, 0.0198974609375, 0.0228271484375, 0.0255126953125, 0.026031494140625, 0.025299072265625, 0.030242919921875, 0.030487060546875, 0.029571533203125, 0.02880859375, 0.02398681640625, 0.029266357421875, 0.02618408203125, 0.026947021484375, 0.022216796875, 0.022247314453125, 0.022552490234375, 0.014373779296875, 0.011444091796875, 0.011444091796875, 0.012115478515625, 0.00823974609375, 0.01446533203125, 0.008636474609375, 0.00726318359375, 0.007720947265625, 0.010406494140625, 0.008758544921875, 0.00848388671875, 0.01226806640625, 0.009368896484375, 0.00732421875, -0.000823974609375, 0.00152587890625, 0.003631591796875, 0.00640869140625, 0.015655517578125, 0.0234375, 0.015960693359375, 0.010955810546875, 0.01055908203125, 0.009185791015625, 0.00994873046875, 0.016632080078125, 0.01751708984375, 0.015411376953125, 0.0157470703125, 0.0189208984375, 0.015167236328125, 0.009735107421875, 0.019439697265625, 0.024169921875, 0.02508544921875, 0.022308349609375, 0.020111083984375, 0.02056884765625, 0.018035888671875, 0.02093505859375, 0.018280029296875, 0.0152587890625, 0.0185546875, 0.01220703125, 0.01251220703125, 0.01544189453125, 0.01629638671875, 0.017120361328125, 0.01385498046875, 0.020416259765625, 0.017181396484375, 0.015960693359375, 0.01318359375, 0.009796142578125, 0.008148193359375, 0.01165771484375, 0.014892578125, 0.01531982421875, 0.013275146484375, 0.01507568359375, 0.0140380859375, 0.011993408203125, 0.0147705078125, 0.017547607421875, 0.013702392578125, 0.014678955078125, 0.014404296875, 0.0152587890625, 0.0140380859375, 0.01116943359375, 0.012176513671875, 0.009674072265625, 0.013153076171875, 0.013397216796875, 0.005462646484375, 0.011749267578125, 0.016021728515625, 0.010101318359375, 0.008819580078125, -0.000396728515625, 0.004852294921875, 0.000457763671875, 0.002838134765625, 0.0035400390625, -0.003662109375, 0.005950927734375, 0.00018310546875, 0.0047607421875, 0.0089111328125, 0.010345458984375, 0.005645751953125, 0.00897216796875, 0.009552001953125, 0.014862060546875, 0.012420654296875, 0.00762939453125, 0.009918212890625, 0.01318359375, 0.013824462890625, 0.01019287109375, 0.01519775390625, 0.018829345703125, 0.020782470703125, 0.022491455078125, 0.02142333984375, 0.01995849609375, 0.013580322265625, 0.01446533203125, 0.0179443359375, 0.012298583984375, 0.014556884765625, 0.01953125, 0.015777587890625, 0.017059326171875, 0.01171875, 0.01025390625, 0.020660400390625, 0.0185546875, 0.02239990234375, 0.026336669921875, 0.019989013671875, 0.01690673828125, 0.01507568359375, 0.0186767578125, 0.014434814453125, 0.01007080078125, 0.01788330078125, 0.016387939453125, 0.018280029296875, 0.016143798828125, 0.01678466796875, 0.012939453125, 0.014251708984375, 0.014923095703125, 0.01190185546875, 0.009674072265625, 0.014251708984375, 0.015106201171875, 0.008392333984375, 0.008544921875, 0.008514404296875, 0.011932373046875, 0.0032958984375, 0.002655029296875, 0.008544921875, 0.006622314453125, 0.012176513671875, 0.00640869140625, 0.008026123046875, 0.0126953125, 0.01043701171875, 0.003570556640625, 0.000457763671875, 0.001495361328125, 0.001190185546875, 0.0052490234375, 0.007659912109375, 0.00634765625, 0.003997802734375, 0.004150390625, 0.00885009765625, 0.00103759765625, 0.003936767578125, 0.00653076171875, 0.0006103515625, -0.000213623046875, 0.000579833984375, -0.001922607421875, 0.00189208984375, 0.002044677734375, 0.00689697265625, 0.005950927734375, 0.008514404296875, 0.010772705078125, 0.00347900390625, 0.008026123046875, 0.005218505859375, 0.005218505859375, 0.004669189453125, 0.011871337890625, 0.01348876953125, 0.015655517578125, 0.010223388671875, 0.0086669921875, 0.0128173828125, 0.0155029296875, 0.022369384765625, 0.018524169921875]
  out "WAVLoopTime":u32(graph)=555
  out "SkippedFrames":i32
  out "FrameCount":i32=1264
  out "AVILoopTime":u32(graph)=37
  out "AVIImage":T6(plugin-control)
  out "BufferNumber":u32=2527
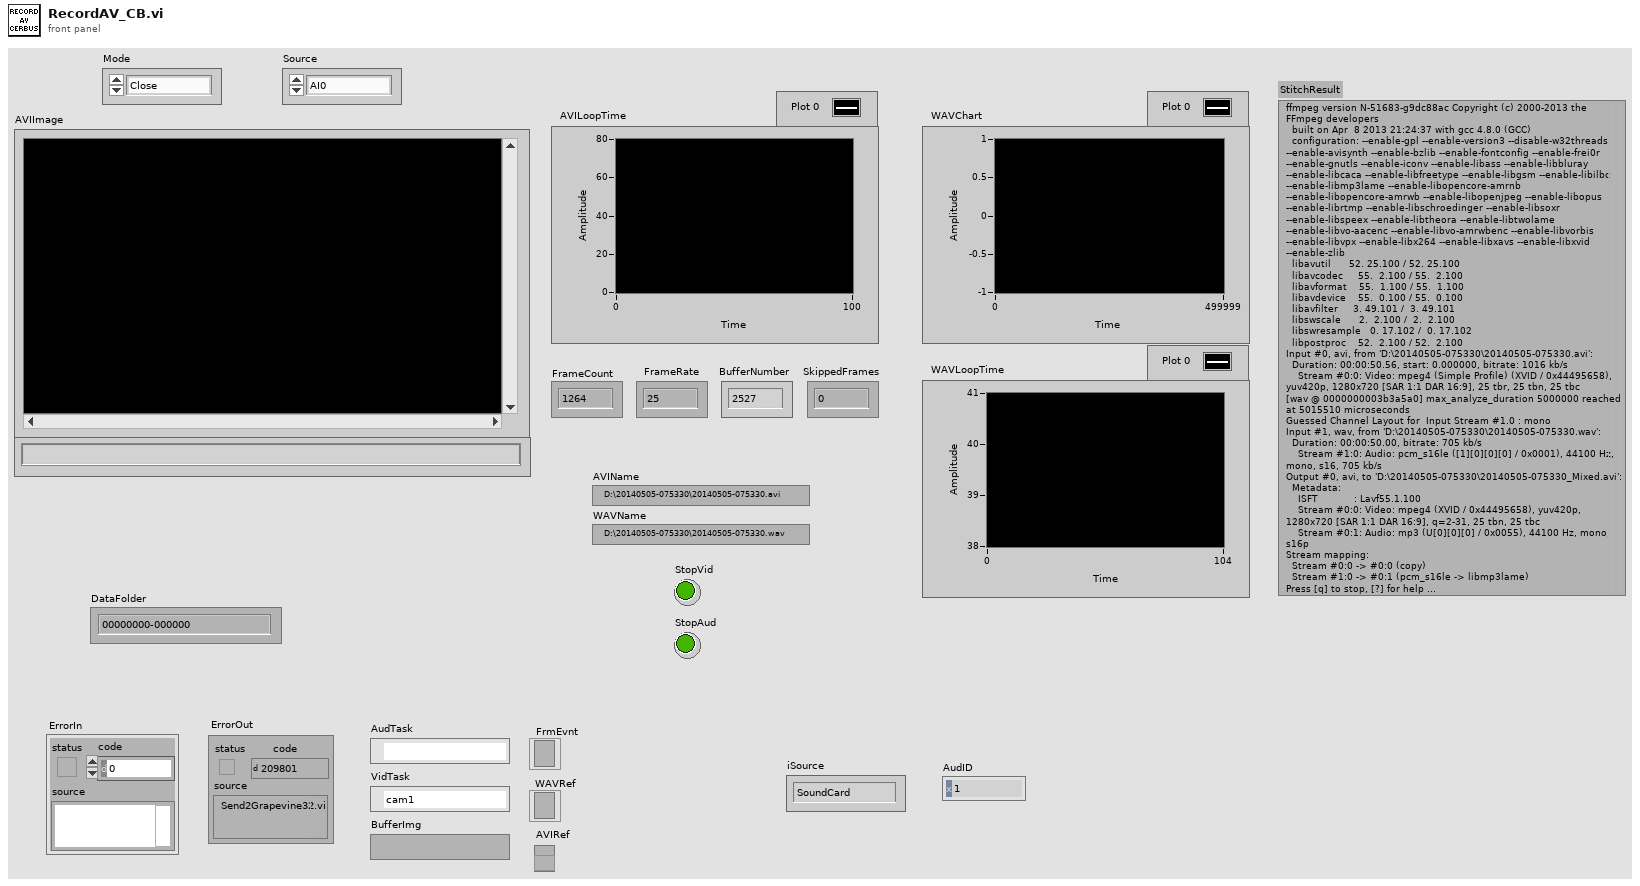
[diagram p1: front panel]
types:
  T1 = typedef "Sound Input Task ID.ctl" = u32
  T2 = enum16{"Initialize", "Start", "Run", "Stop", "Close"}
  T3 = typedef "IMAQdx.ctl" = refnum<k21>
  T4 = typedef "Sound File Refnum.ctl" = refnum<file>
  T5 = typedef "IMAQ AVI2 Refnum.ctl" = refnum<k20>
  T6 = typedef "IMAQ Image.ctl" = refnum<image>
  T7 = enum16{"Initialize", "String", "Start", "Stop", "Close"}
  T8 = typedef "Sound Data Format.ctl" = cluster{"sample rate (S/s)":dbl, "number of channels":i32, "bits per sample":i32}
  T9 = typedef "NI_Vision_Acquisition_Software.lvlib/IMAQdx Acquisition Mode.ctl" = enum32{"One Shot", "Continuous"}
  T10 = typedef "NI_Vision_Acquisition_Software.lvlib/IMAQdx Buffer Number Mode.ctl" = enum32{"Next", "Last", "Buffer Number"}
  T11 = typedef "Sampling Mode.ctl" = i32
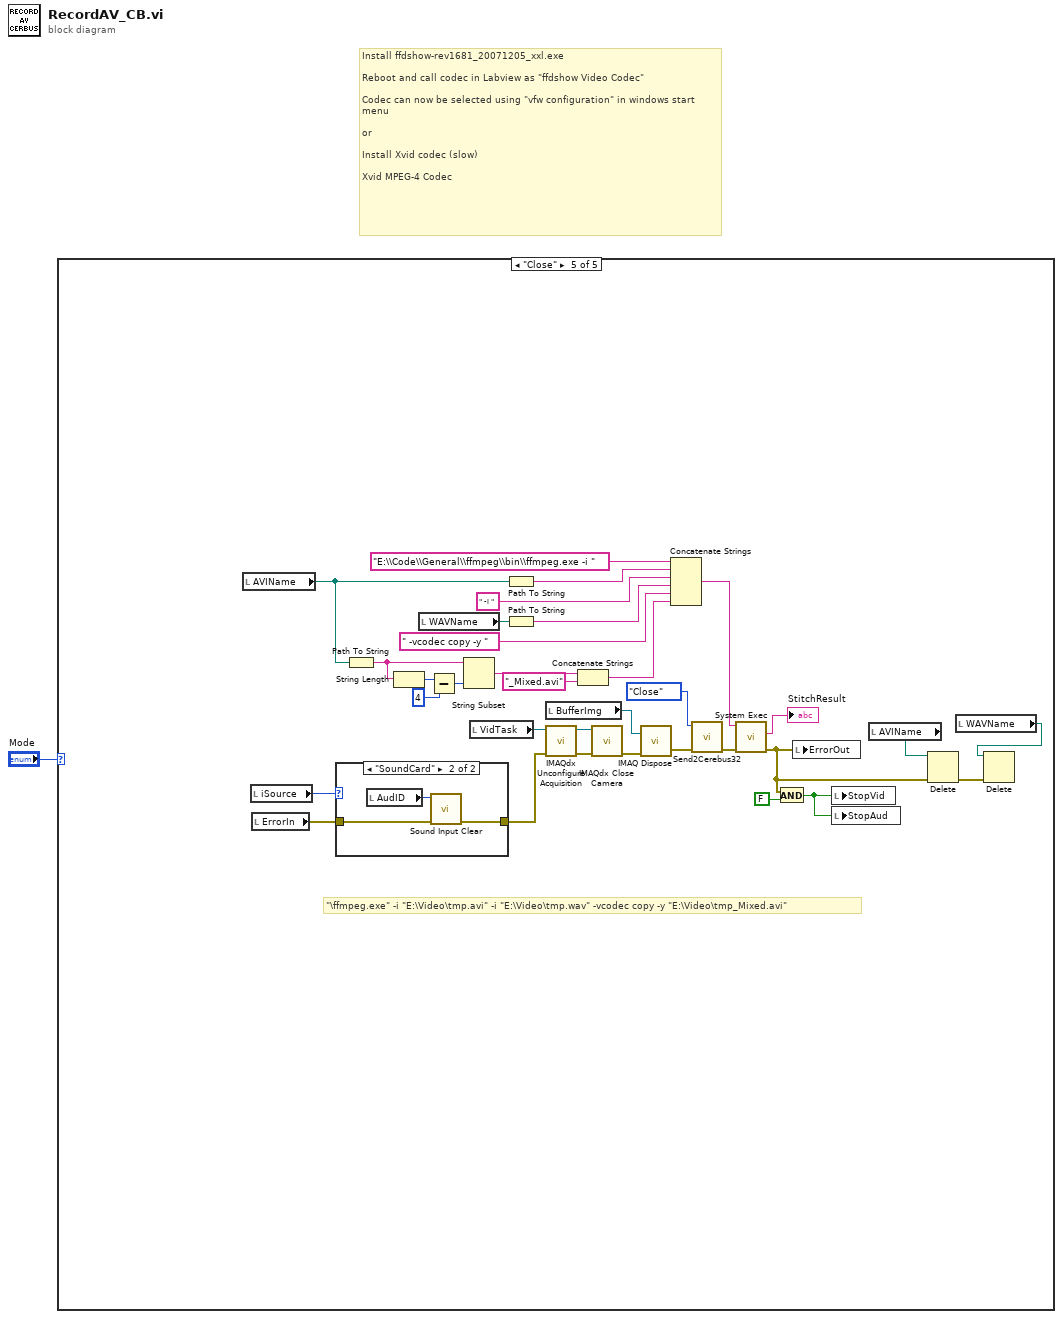
[diagram p0: block diagram]
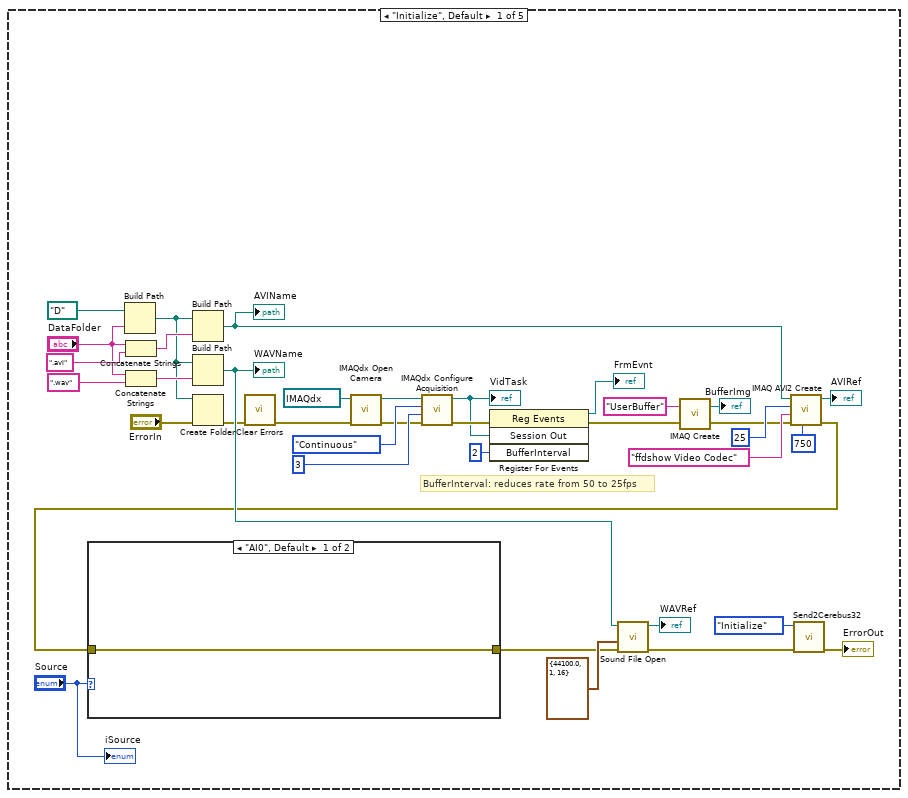
[diagram p2: hidden frame]
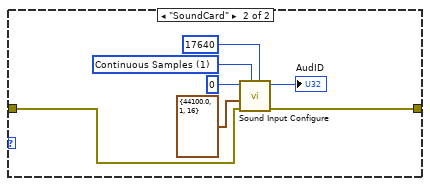
[diagram p3: hidden frame]
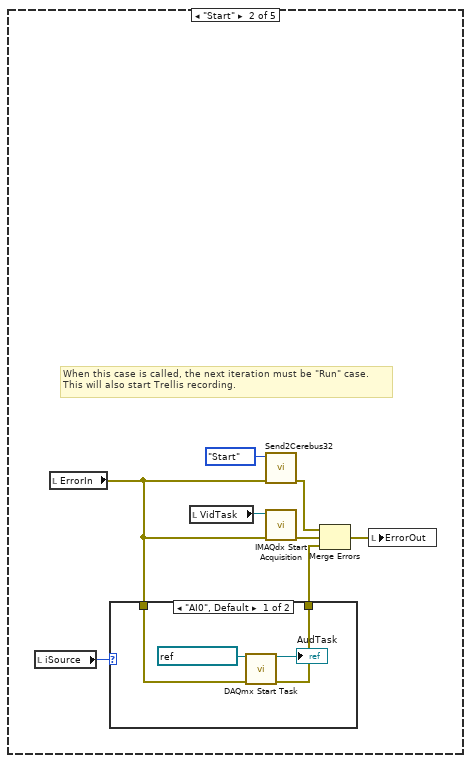
[diagram p4: hidden frame]
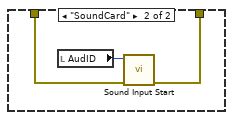
[diagram p5: hidden frame]
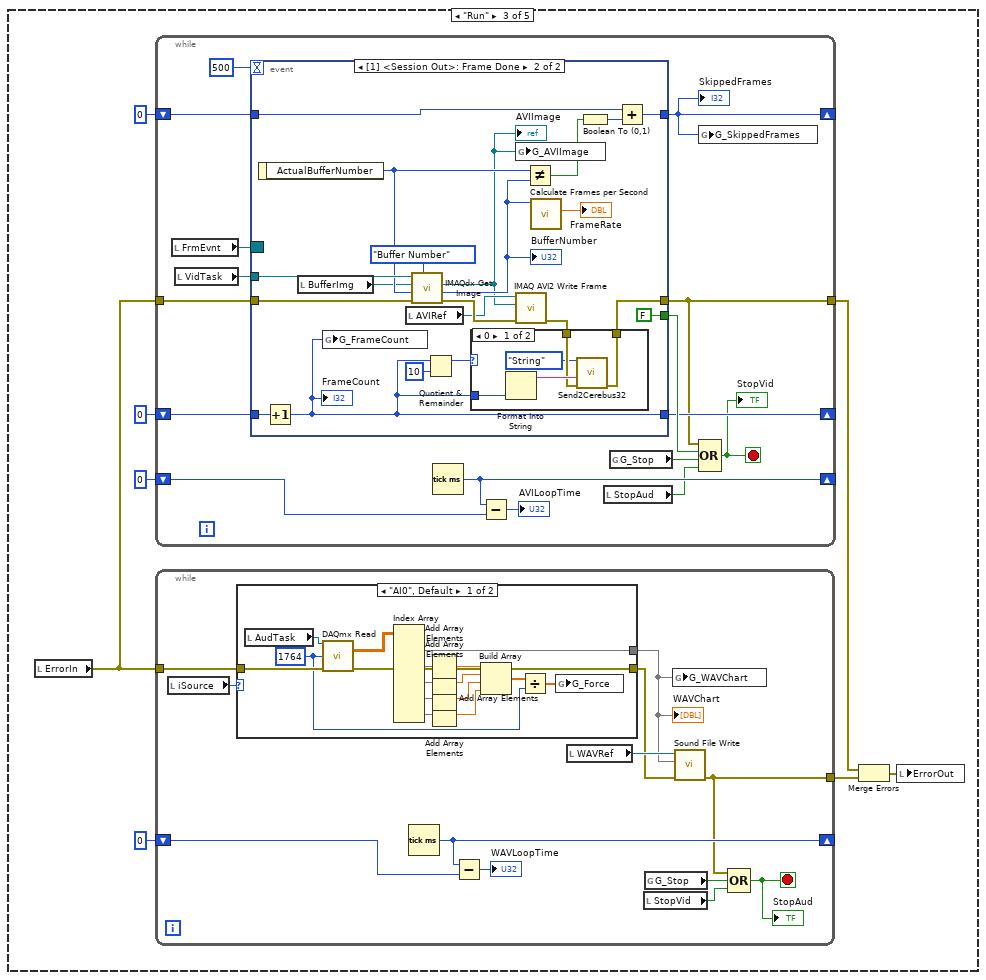
[diagram p6: hidden frame]
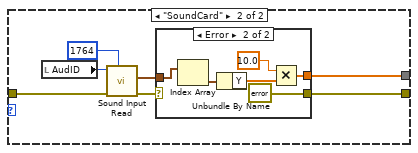
[diagram p7: hidden frame]
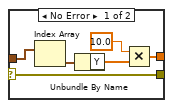
[diagram p8: hidden frame]
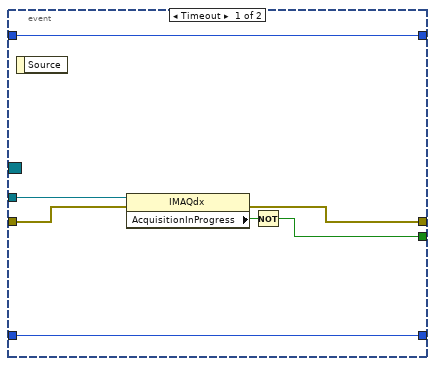
[diagram p9: hidden frame]
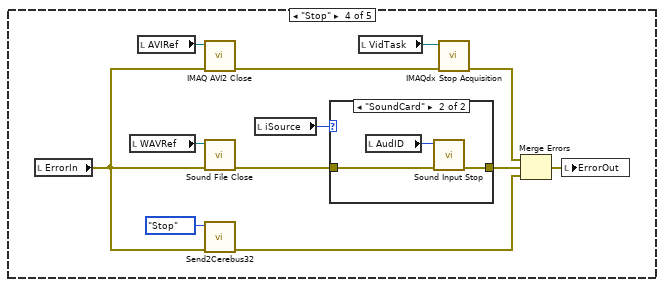
[diagram p11: hidden frame]
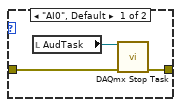
[diagram p12: hidden frame]
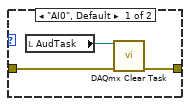
[diagram p13: hidden frame]
diagram:
  # "Install ffdshow-rev1681_20071205_xxl.exe\n\nReboot and call codec in Labview as \"ffdshow Video Codec\"\n\nCodec can now be selected using \"vfw configuration\" in windows start menu\n\nor\n\nInstall Xvid codec (slow)\n\nXvid MPEG-4 Codec"
  n1 = case shown="\"Close\"" "Mode" {
    frame "Initialize", Default {
      # "BufferInterval: reduces rate from 50 to 25fps"
      n2 = Build Path(base path=path "D:/", name or relative path="DataFolder") -> (appended path=w7:path)
      n3 = Concatenate Strings("DataFolder", ".avi" ("string")) -> (w29:string)
      n4 = Concatenate Strings("DataFolder", ".wav" ("string")) -> (w30:string)
      n5 = Build Path(base path=w7, name or relative path=w29) -> (appended path=w31:path)
      "AVIName" <- w31
      n6 = Build Path(base path=w7, name or relative path=w30) -> (appended path=w32:path)
      "WAVName" <- w32
      n7 = Create Folder(path (use dialog)=w7, error in="ErrorIn") -> (error out=w5:errorcluster)  [unwired: 1 in, 2 out]
      n8 = call <vilib>:"Clear Errors.vi"("error in (no error)"=w5) -> ("error out"=w4:errorcluster)  [unwired: 6 in]
      n9 = call <vilib>:"IMAQdx Open Camera.vi"("error in"=w4, "Session In"=T3 "cam1") -> ("error out"=w15:errorcluster, "Session Out"=w14:T3)  [unwired: 1 in, 7 out]
      n10 = call <vilib>:"IMAQdx Configure Acquisition.vi"("error in"=w15, "Number of Buffers"=u32 3 ("InternalBufferNumber"), "Continuous?"=IMAQdx_Acquisition_Mode."Continuous", "Session In"=w14) -> ("error out"=w18:errorcluster, "Session Out"=w12:T3)  [unwired: 6 out]
      "VidTask" <- w12
      n11 = register-events(error in=w18, w12, u32 2 ("BufferInterval")) -> (reference out=→"FrmEvnt":refnum<event-registration>, error out=w22:errorcluster)  [unwired: 1 in]
      n12 = call "IMAQ Create"("Image Name"="UserBuffer", "error in (no error)"=w22) -> ("New Image"=→"BufferImg":T6, "error out"=w23:errorcluster)  [unwired: 2 in, 1 out]
      n13 = call "IMAQ AVI2 Create"("Quality"=750, "error in (no error)"=w23, "Codec"="ffdshow Video Codec", "Frames Per Second"=u32 25, "AVI Path"=w31) -> ("error out"=w24:errorcluster, "AVI Refnum"=→"AVIRef":T5)  [unwired: 5 in]
      n14 = case shown="\"AI0\", Default" "Source" {
        tunnel: w24 -> [w39 w44]
        tunnel: [w39 w43] -> w10
        frame "AI0", Default {
        }
        frame "SoundCard" {
          w41 = T11 1 items=["Finite Samples", "Continuous Samples"] ("sample mode")
          n15 = call <vilib>:"Sound Input Configure.vi"("number of samples/ch"=17640, "sample mode"=w41, "error in (no error)"=w44, "sound format"=T8 {"sample rate (S/s)"=44100.0, "number of channels"=1, "bits per sample"=16}, "device ID"=u32 0) -> ("error out"=w43:errorcluster, "task ID"=→"AudID":T1)  [unwired: 5 in]
        }
      }
      n16 = call-poly <vilib>:"Sound File Open.vi"("error in (no error)"=w10, "sound format"=T8 {"sample rate (S/s)"=44100.0, "number of channels"=1, "bits per sample"=16}, "path"=w32) -> ("error out"=w38:errorcluster, "sound file refnum"=→"WAVRef":T4)  [unwired: 7 in]
      n17 = call "Send2Cerebus32.vi"("ErrorIn"=w38, "Mode"=T7."Initialize") -> ("ErrorOut"=→"ErrorOut":errorcluster)  [unwired: 5 in]
      "iSource" <- "Source"
    }
    frame "Start" {
      # "When this case is called, the next iteration must be \"Run\" case.\nThis will also start Trellis recording."
      n18 = local read "iSource"() -> (w47:enum16{"AI0", "SoundCard"})
      n19 = local read "ErrorIn"() -> (w49:errorcluster)
      n20 = case shown="\"AI0\", Default" w47 {
        tunnel: w49 -> [w58 w60]
        tunnel: [w57 w59] -> w48
        frame "AI0", Default {
          n21 = call <vilib>:"DAQmx Start Task.vi"("task/channels in"=refnum<k21> "aud_force", "error in"=w58) -> ("task out"=→"AudTask":refnum<k21>, "error out"=w57:errorcluster)  [unwired: 12 in]
        }
        frame "SoundCard" {
          n22 = local read "AudID"() -> (w61:T1)
          n23 = call <vilib>:"Sound Input Start.vi"("error in (no error)"=w60, "task ID"=w61) -> ("error out"=w59:errorcluster)  [unwired: 8 in, 1 out]
        }
      }
      n24 = local read "VidTask"() -> (w53:T3)
      n25 = call "Send2Cerebus32.vi"("ErrorIn"=w49, "Mode"=T7."Start") -> ("ErrorOut"=w52:errorcluster)  [unwired: 5 in]
      n26 = call <vilib>:"IMAQdx Start Acquisition.vi"("error in"=w49, "Session In"=w53) -> ("error out"=w51:errorcluster)  [unwired: 9 out]
      n27 = Merge Errors(w52, w51, w48) -> (w50:errorcluster)
      n28 = local write "ErrorOut"(w50) -> ()
    }
    frame "Run" {
      n29 = local read "ErrorIn"() -> (w64:errorcluster)
      n30 = while {
        tunnel: w64 -> [w132]
        tunnel: [w123] -> w67
        shift-right: [w129] -> _
        shift-left: u32 0 ("millisecond timer value") -> [w128]
        shift-right: [w125] -> _
        shift-left: 0 -> [w126]
        shift-right: [w118] -> _
        shift-left: 0 -> [w124]
        stop <- w122 stop-if-true
        n31 = local read "FrmEvnt"() -> (w120:refnum<event-registration>)
        n32 = local read "VidTask"() -> (w117:T3)
        n33 = event shown="[1] <Session Out>: Frame Done" {
          selector: w120 -> [_ _]
          dyn-events: _ -> [_ _]
          timeout: 500 -> [_ _]
          tunnel: w117 -> [w139 w160]
          tunnel: w132 -> [w138 w159]
          tunnel: [w137 w142] -> w123
          tunnel: [w135 FALSE] -> w130
          tunnel: w126 -> [w134 w153]
          tunnel: [w134 w140] -> w125
          tunnel: w124 -> [w133 w150]
          tunnel: [w133 w149] -> w118
          event Timeout {
            n34 = event-data() -> ()  [unwired: 2 out]
            n35 = property class="IMAQdx"(reference=w139, error in=w138) -> (error out=w137:errorcluster, "AcquisitionInProgress"=w136:bool)  [unwired: 1 out]
            n36 = Not(x=w136) -> (.not. x?=w135:bool)
          }
          event event #0x0 {
            n37 = event-data() -> ("ActualBufferNumber"=w157:u32)  [unwired: 1 out]
            n38 = Increment(x=w153) -> (x+1=w140:i32)
            "FrameCount" <- w140
            n39 = local read "BufferImg"() -> (w147:T6)
            n40 = global write "Globals.vi" "G_FrameCount"(w140) -> ()
            n41 = local read "AVIRef"() -> (w146:T5)
            n42 = call <vilib>:"IMAQdx Get Image.vi"("Buffer Number Mode (Next)"=IMAQdx_Buffer_Number_Mode."Buffer Number" ("Buffer Number Mode"), "error in"=w159, "Buffer Number In"=w157, "Image In"=w147, "Session In"=w160) -> ("error out"=w156:errorcluster, "Buffer Number Out"=w154:u32, "Image Out"=w141:T6)  [unwired: 4 out]
            "BufferNumber" <- w154
            "AVIImage" <- w141
            n43 = Quotient & Remainder(x=w140, y=10) -> (x-y*floor(x/y)=w144:i32)  [unwired: 1 out]
            n44 = global write "Globals.vi" "G_AVIImage"(w141) -> ()
            n45 = call "IMAQ AVI2 Write Frame"("error in (no error)"=w156, "Image"=w141, "AVI Refnum"=w146) -> ("error out"=w143:errorcluster)  [unwired: 6 in, 2 out]
            n46 = case shown="0" w144 {
              tunnel: w140 -> [w165 _]
              tunnel: w143 -> [w163 w166]
              tunnel: [w162 w166] -> w142
              frame 0 {
                n47 = Format Into String(w165) -> (resulting string=w164:string)  [unwired: 3 in, 1 out]
                n48 = call "Send2Cerebus32.vi"("ErrorIn"=w163, "String"=w164, "Mode"=T7."String") -> ("ErrorOut"=w162:errorcluster)  [unwired: 4 in]
              }
              frame 1, Default {
              }
            }
            n49 = Not Equal?(x=w157, y=w154) -> (x != y?=w152:bool)
            n50 = call <vilib>:"Calculate Frames per Second.vi"("Buffer Number"=w154) -> ("Processed Frames/s"=→"FrameRate":dbl)  [unwired: 8 in, 2 out]
            n51 = Boolean To (0,1)(Boolean=w152) -> (0, 1=w151:i16)
            n52 = Add(x=w150, y=w151) -> (x+y=w149:i32)
          }
        }
        "SkippedFrames" <- w118
        n53 = Tick Count (ms)() -> (millisecond timer value=w129:u32)
        n54 = Subtract(x=w129, y=w128) -> (x-y=→"AVILoopTime":u32)
        n55 = local read "StopAud"() -> (w121:bool)
        n56 = global read "Globals.vi" "G_Stop"() -> (w119:bool)
        n57 = global write "Globals.vi" "G_SkippedFrames"(w118) -> ()
        n58 = Compound Arithmetic op=OR(w123, w130, w119, w121) -> (w122:bool)
        "StopVid" <- w122
      }
      n59 = while {
        tunnel: w64 -> [w71]
        tunnel: [w78] -> w66
        shift-right: [w81] -> _
        shift-left: u32 0 ("millisecond timer value") -> [w80]
        stop <- w77 stop-if-true
        n60 = local read "iSource"() -> (w70:enum16{"AI0", "SoundCard"})
        n61 = case shown="\"AI0\", Default" w70 {
          tunnel: w71 -> [w97 w104]
          tunnel: [w96 w98] -> w72
          tunnel: [w94 w100] -> w73
          frame "AI0", Default {
            w82 = 1764 ("number of samples per channel")
            n62 = local read "AudTask"() -> (w95:refnum<k21>)
            n63 = call-poly <vilib>:"DAQmx Read.vi"("task/channels in"=w95, "number of samples per channel"=w82, "error in"=w97) -> ("data"=w93:dbl[][], "error out"=w96:errorcluster)  [unwired: 10 in, 1 out]
            n64 = Index Array(array=w93) -> (element #1=w94:dbl[], element #2=w92:dbl[], element #3=w91:dbl[], element #4=w90:dbl[], element #5=w89:dbl[])  [unwired: 10 in]
            n65 = Add Array Elements(numeric array=w92) -> (sum=w87:dbl)
            n66 = Add Array Elements(numeric array=w91) -> (sum=w88:dbl)
            n67 = Add Array Elements(numeric array=w90) -> (sum=w86:dbl)
            n68 = Add Array Elements(numeric array=w89) -> (sum=w85:dbl)
            n69 = Build Array(w87, w88, w86, w85) -> (w84:dbl[])
            n70 = Divide(x=w84, y=w82) -> (x/y=w83:dbl[])
            n71 = global write "Globals.vi" "G_Force"(w83) -> ()
          }
          frame "SoundCard" {
            n72 = local read "AudID"() -> (w101:T1)
            n73 = call-poly <vilib>:"Sound Input Read.vi"("number of samples/ch"=1764 ("number of samples per channel"), "error in (no error)"=w104, "task ID"=w101) -> ("error out"=w99:errorcluster, "data"=w102:waveform(sgl)[])  [unwired: 6 in, 1 out]
            n74 = case shown="Error" w99 {
              selector: w99 -> [w105 _]
              tunnel: w102 -> [w110 w113]
              tunnel: [w109 w112] -> w100
              tunnel: [w105 errorcluster {"status"=FALSE, "code"=0, "source"=""} ("error IO")] -> w98
              frame No Error {
                n75 = Index Array(array=w110) -> (element=w108:waveform(sgl))  [unwired: 1 in]
                n76 = Unbundle By Name(w108) -> ("Y"=w107:sgl[])
                n77 = Multiply(x=10.0, y=w107) -> (x*y=w109:dbl[])
              }
              frame Error {
                n78 = Index Array(array=w113) -> (element=w116:waveform(sgl))  [unwired: 1 in]
                n79 = Unbundle By Name(w116) -> ("Y"=w115:sgl[])
                n80 = Multiply(x=10.0, y=w115) -> (x*y=w112:dbl[])
              }
            }
          }
        }
        "WAVChart" <- w73
        n81 = Tick Count (ms)() -> (millisecond timer value=w81:u32)
        n82 = Subtract(x=w81, y=w80) -> (x-y=→"WAVLoopTime":u32)
        n83 = local read "WAVRef"() -> (w75:T4)
        n84 = local read "StopVid"() -> (w76:bool)
        n85 = global read "Globals.vi" "G_Stop"() -> (w74:bool)
        n86 = global write "Globals.vi" "G_WAVChart"(w73) -> ()
        n87 = call-poly <vilib>:"Sound File Write.vi"("error in (no error)"=w72, "data"=w73, "sound file refnum"=w75) -> ("error out"=w78:errorcluster)  [unwired: 7 in, 1 out]
        n88 = Compound Arithmetic op=OR(w78, w74, w76) -> (w77:bool)
        "StopAud" <- w77
      }
      n89 = Merge Errors(w67, w66) -> (w65:errorcluster)
      n90 = local write "ErrorOut"(w65) -> ()
    }
    frame "Stop" {
      n91 = local read "ErrorIn"() -> (w170:errorcluster)
      n92 = local read "WAVRef"() -> (w177:T4)
      n93 = local read "AVIRef"() -> (w176:T5)
      n94 = call "IMAQ AVI2 Close"("error in (no error)"=w170, "AVI Refnum"=w176) -> ("error out"=w174:errorcluster)  [unwired: 9 in]
      n95 = call <vilib>:"Sound File Close.vi"("error in (no error)"=w170, "sound file refnum"=w177) -> ("error out"=w175:errorcluster)  [unwired: 9 in]
      n96 = call "Send2Cerebus32.vi"("ErrorIn"=w170, "Mode"=T7."Stop") -> ("ErrorOut"=w168:errorcluster)  [unwired: 5 in]
      n97 = local read "iSource"() -> (w167:enum16{"AI0", "SoundCard"})
      n98 = case shown="\"SoundCard\"" w167 {
        tunnel: w175 -> [w180 w183]
        tunnel: [w179 w182] -> w172
        frame "AI0", Default {
          n99 = local read "AudTask"() -> (w181:refnum<k21>)
          n100 = call <vilib>:"DAQmx Stop Task.vi"("task/channels in"=w181, "error in"=w180) -> ("error out"=w179:errorcluster)  [unwired: 12 in, 1 out]
        }
        frame "SoundCard" {
          n101 = local read "AudID"() -> (w184:T1)
          n102 = call <vilib>:"Sound Input Stop.vi"("error in (no error)"=w183, "task ID"=w184) -> ("error out"=w182:errorcluster)  [unwired: 8 in, 1 out]
        }
      }
      n103 = local read "VidTask"() -> (w178:T3)
      n104 = call <vilib>:"IMAQdx Stop Acquisition.vi"("error in"=w174, "Session In"=w178) -> ("error out"=w173:errorcluster)  [unwired: 9 out]
      n105 = Merge Errors(w173, w172, w168) -> (w171:errorcluster)
      n106 = local write "ErrorOut"(w171) -> ()
    }
    frame "Close" {
      # "\"\\ffmpeg.exe\" -i \"E:\\Video\\tmp.avi\" -i \"E:\\Video\\tmp.wav\" -vcodec copy -y \"E:\\Video\\tmp_Mixed.avi\""
      n107 = local read "AVIName"() -> (w192:path)
      n108 = local read "iSource"() -> (w189:enum16{"AI0", "SoundCard"})
      n109 = local read "ErrorIn"() -> (w199:errorcluster)
      n110 = case shown="\"SoundCard\"" w189 {
        tunnel: w199 -> [w219 w222]
        tunnel: [w218 w221] -> w197
        frame "AI0", Default {
          n111 = local read "AudTask"() -> (w220:refnum<k21>)
          n112 = call <vilib>:"DAQmx Clear Task.vi"("task in"=w220, "error in"=w219) -> ("error out"=w218:errorcluster)  [unwired: 13 in]
        }
        frame "SoundCard" {
          n113 = local read "AudID"() -> (w223:T1)
          n114 = call <vilib>:"Sound Input Clear.vi"("error in (no error)"=w222, "task ID"=w223) -> ("error out"=w221:errorcluster)  [unwired: 9 in]
        }
      }
      n115 = Path To String(path=w192) -> (string=w193:string)
      n116 = String Length(string=w193) -> (length=w195:i32)
      n117 = local read "WAVName"() -> (w210:path)
      n118 = Subtract(x=w195, y=4) -> (x-y=w194:i32)
      n119 = String Subset(string=w193, length (rest)=w194) -> (substring=w191:string)  [unwired: 1 in]
      n120 = local read "VidTask"() -> (w198:T3)
      n121 = Path To String(path=w192) -> (string=w208:string)
      n122 = Path To String(path=w210) -> (string=w211:string)
      n123 = local read "BufferImg"() -> (w217:T6)
      n124 = call <vilib>:"IMAQdx Unconfigure Acquisition.vi"("error in"=w197, "Session In"=w198) -> ("error out"=w204:errorcluster, "Session Out"=w205:T3)  [unwired: 8 out]
      n125 = Concatenate Strings(w191, "_Mixed.avi" ("string")) -> (w190:string)
      n126 = call <vilib>:"IMAQdx Close Camera.vi"("error in"=w204, "Session In"=w205) -> ("error out"=w206:errorcluster)  [unwired: 9 out]
      n127 = call "IMAQ Dispose"("Image"=w217, "error in (no error)"=w206) -> ("error out"=w203:errorcluster)  [unwired: 4 in]
      n128 = Concatenate Strings("E:\\Code\\General\\ffmpeg\\bin\\ffmpeg.exe -i ", w208, " -i " ("string"), w211, " -vcodec copy -y " ("string"), w190) -> (w214:string)
      n129 = call "Send2Cerebus32.vi"("ErrorIn"=w203, "Mode"=T7."Close") -> ("ErrorOut"=w202:errorcluster)  [unwired: 5 in]
      n130 = call <vilib>:"System Exec.vi"("error in (no error)"=w202, "command line"=w214) -> ("error out"=w188:errorcluster, "standard error"=→"StitchResult":string)  [unwired: 6 in, 2 out]
      n131 = And(x=w188, y=FALSE) -> (x .and. y?=w201:bool)
      n132 = local write "ErrorOut"(w188) -> ()
      n133 = local write "StopVid"(w201) -> ()
      n134 = local write "StopAud"(w201) -> ()
      n135 = local read "AVIName"() -> (w187:path)
      n136 = Delete(path (use dialog)=w187, error in=w188) -> (error out=w186:errorcluster)  [unwired: 3 in, 2 out]
      n137 = local read "WAVName"() -> (w185:path)
      n138 = Delete(path (use dialog)=w185, error in=w186) -> ()  [unwired: 3 in, 3 out]
    }
  }
